vi "ResetTable.vi"(8 "Error In":errorcluster, 11 "Table in":refnum<vi>) -> (0 "Error Out":errorcluster)   [LabVIEW 2017, in "Client.lvlib" / "UI_API.lvlib"]
uses:
  UI_API.lvlib
  <vilib>/Utility/miscctls.llb/LVRowAndColumnTypeDef.ctl
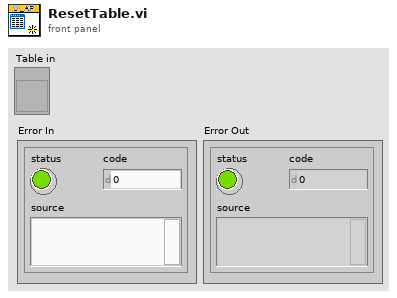
[diagram p1: front panel]
types:
  T1 = typedef "LVRowAndColumnTypeDef.ctl" = cluster{"Row":i32, "Column":i32}
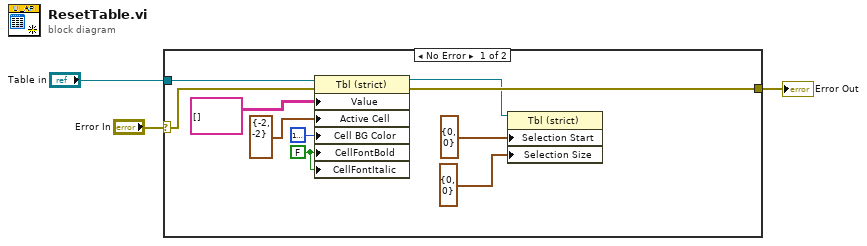
[diagram p0: block diagram]
diagram:
  n1 = case shown="No Error" "Error In" {
    selector: "Error In" -> [w8 w14]
    tunnel: "Table in" -> [w9 _]
    tunnel: [w7 w14] -> w1
    frame No Error {
      w13 = FALSE ("Active Cell:Cell Font:Bold")
      n2 = property class="Tbl (strict)"(reference=w9, error in=w8, "Value"=string[][] [], "Active Cell"=T1 {"Row"=-2, "Column"=-2} ("Active Cell:Active Cell"), "Cell BG Color"=u32 16777225, "CellFontBold"=w13, "CellFontItalic"=w13) -> (reference out=w6:refnum<vi>, error out=w7:errorcluster)
      n3 = property class="Tbl (strict)"(reference=w6, "Selection Start"=T1 {"Row"=0, "Column"=0}, "Selection Size"=T1 {"Row"=0, "Column"=0}) -> ()  [unwired: 1 in, 2 out]
    }
    frame Error {
    }
  }
  "Error Out" <- w1
